vi "TIME（算法1）.vi"() -> ()   [LabVIEW 2017]
panel:
  out "回文质数数量":dbl
  out "回文质数":dbl[](array[numeric])
  out "数值":dbl
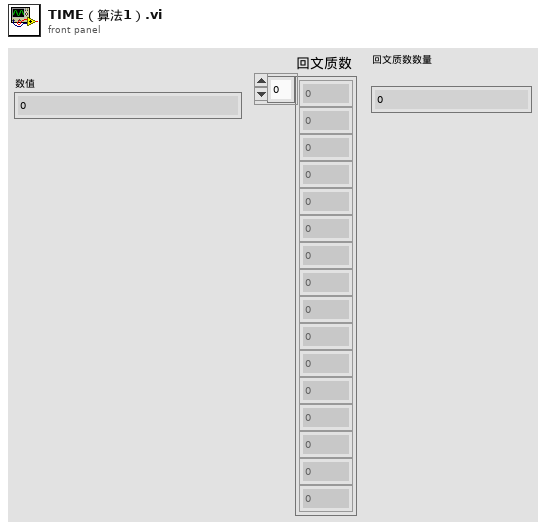
[diagram p1: front panel]
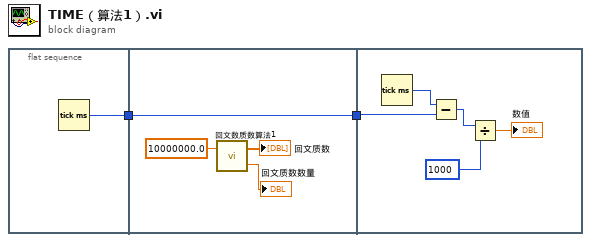
[diagram p0: block diagram]
diagram:
  n1 = flat-sequence {
    tunnel: [w3] -> w1
    tunnel: [w7] -> w2
    tunnel: w1 -> [w7]
    tunnel: w2 -> [w9]
    frame #0 {
      n2 = Tick Count (ms)() -> (millisecond timer value=w3:u32)
    }
    frame #1 {
      n3 = call "回文数质数算法1.vi"("上限"=10000000.0) -> ("回文质数数量"=→"回文质数数量":dbl, "回文质数"=→"回文质数":dbl[])  [unwired: 1 in]
    }
    frame #2 {
      n4 = Tick Count (ms)() -> (millisecond timer value=w8:u32)
      n5 = Subtract(x=w8, y=w9) -> (x-y=w12:u32)
      n6 = Divide(x=w12, y=u32 1000) -> (x/y=→"数值":dbl)
    }
  }
